vi "DigitalInput Reservations.vi"(3 "Reset":bool, 5 "Line":tag) -> (0 "Exit code":T1, 1 "Index assigned":i32, 2 "DigitalInput lines":tag[](array[tag]))   [LabVIEW 2015]
doc: "Attempt to reserve a line as a digital input. This also returns a list of lines that have been previously reserved.\n\nAs a Device developer, just call this with the line you want to add, check that the exit code is good, and save the assigned index.\n\nAs a Rack developer, remember to reset the reservations list before Device initialization and then call it with an empty line afterwards to get the list of digital output lines."
uses:
  Typedefs/Reservation exit codes.ctl
  <vilib>/Utility/error.llb/DialogType.ctl
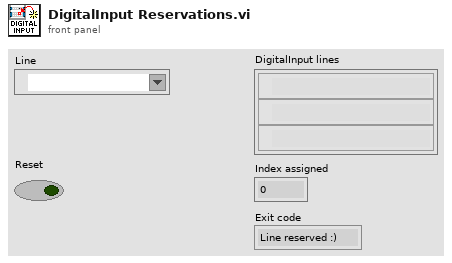
[diagram p1: front panel]
types:
  T1 = typedef "Reservation exit codes.ctl" = enum16{"Line reserved :)", "List reset.", "Empty line!", "Bad line!", "Already reserved!", "Timestamp conflict!", "Timestamp empty."}
  T2 = typedef "DialogType.ctl" = u16
  T3 = enum16{"Analog input", "Analog output", "Digital input", "Digital output", "Counter input", "Counter output"}
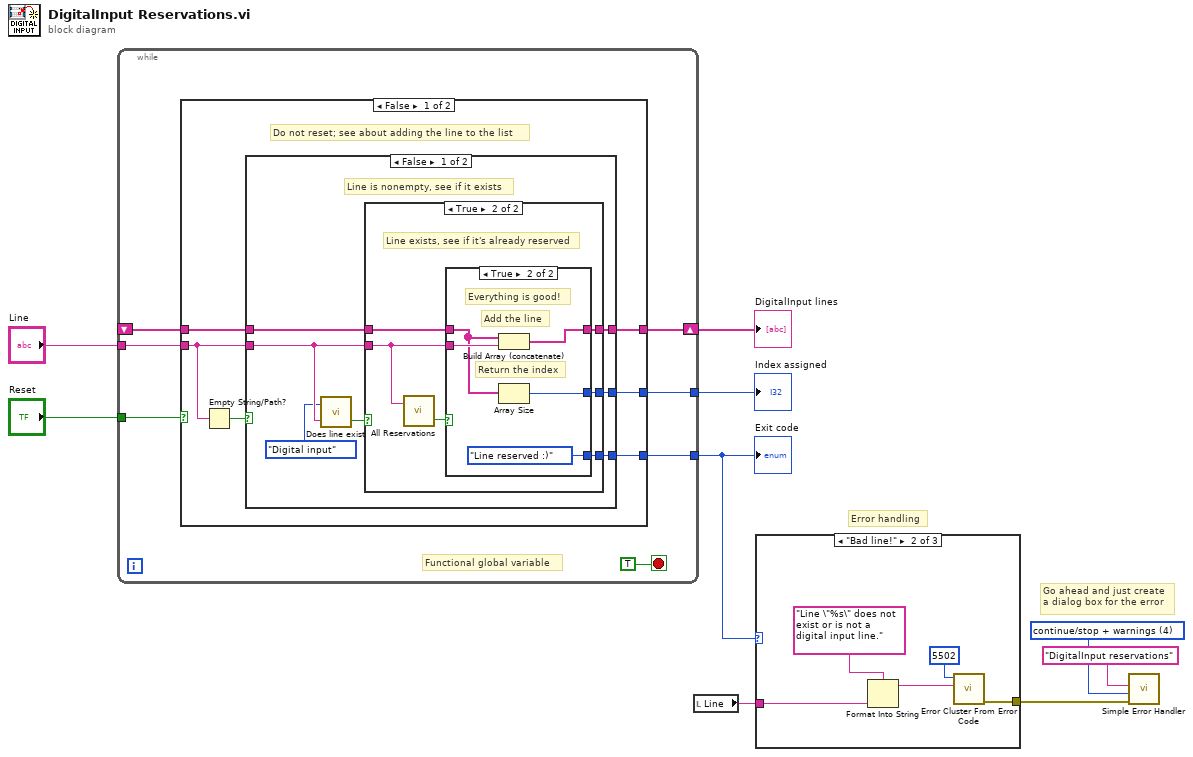
[diagram p0: block diagram]
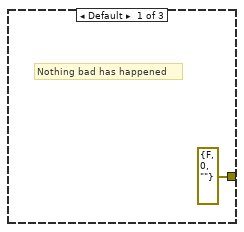
[diagram p2: hidden frame]
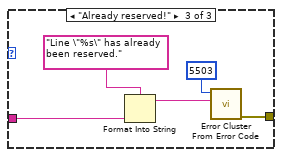
[diagram p3: hidden frame]
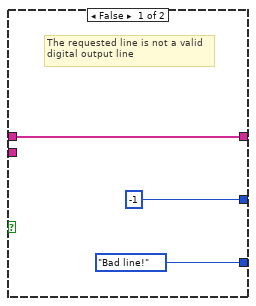
[diagram p4: hidden frame]
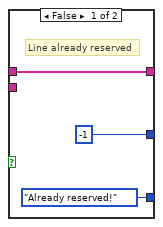
[diagram p5: hidden frame]
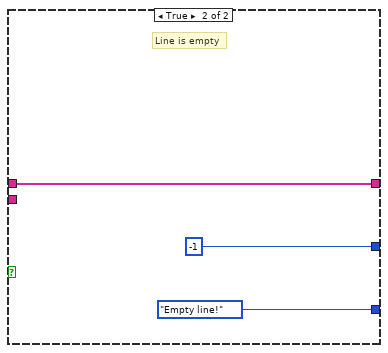
[diagram p6: hidden frame]
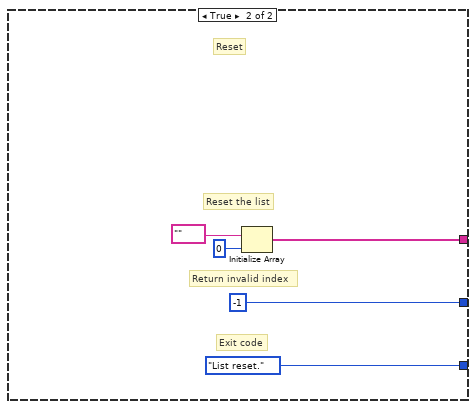
[diagram p7: hidden frame]
diagram:
  w4 = T2 4 items=["no dialog", "OK message", "continue or stop message", "OK message + warnings", "continue/stop + warnings"] ("type of dialog (OK msg:1)")
  # "Error handling"
  # "Go ahead and just create\na dialog box for the error"
  n1 = while {
    tunnel: [w16] -> w2
    tunnel: "Reset" -> [w15]
    shift-right: [w14] -> w9
    shift-left: _ -> [w12]
    tunnel: "Line" -> [w11]
    tunnel: [w10] -> w7
    stop <- TRUE ("stop") stop-if-true
    # "Functional global variable"
    n2 = case shown="False" w15 {
      tunnel: [w19 Reservation_exit_codes."List reset." ("Exit code")] -> w16
      tunnel: [w22 w53] -> w14
      tunnel: w12 -> [w21 _]
      tunnel: w11 -> [w17 _]
      tunnel: [w20 -1 ("Index assigned")] -> w10
      frame False {
        # "Do not reset; see about adding the line to the list"
        n3 = Empty String/Path?(string/path=w17) -> (empty?=w18:bool)
        n4 = case shown="False" w18 {
          tunnel: [w29 w49] -> w22
          tunnel: w21 -> [w28 w49]
          tunnel: [w27 -1] -> w20
          tunnel: [w26 Reservation_exit_codes."Empty line!" ("Exit code")] -> w19
          tunnel: w17 -> [w24 _]
          frame False {
            # "Line is nonempty, see if it exists"
            n5 = call "Does line exist.vi"("Line to look for"=w24, "Line type"=T3."Digital input") -> ("Does line exist?"=w25:bool)  [unwired: 1 out]
            n6 = case shown="True" w25 {
              tunnel: [w32 w38] -> w29
              tunnel: w28 -> [w32 w37]
              tunnel: [-1 w36] -> w27
              tunnel: [Reservation_exit_codes."Bad line!" ("Exit code") w35] -> w26
              tunnel: w24 -> [_ w33]
              frame False {
                # "The requested line is not a valid\ndigital output line"
              }
              frame True {
                # "Line exists, see if it's already reserved"
                n7 = call "All Reservations.vi"("Line to add"=w33) -> ("Line added?"=w34:bool)  [unwired: 1 in, 1 out]
                n8 = case shown="True" w34 {
                  tunnel: w37 -> [w41 w44]
                  tunnel: [w41 w46] -> w38
                  tunnel: w33 -> [_ w45]
                  tunnel: [-1 w43] -> w36
                  tunnel: [Reservation_exit_codes."Already reserved!" ("Exit code") Reservation_exit_codes."Line reserved :)" ("Exit code")] -> w35
                  frame False {
                    # "Line already reserved"
                  }
                  frame True {
                    # "Everything is good!"
                    # "Return the index"
                    # "Add the line"
                    n9 = Build Array (concatenate)(w44, w45) -> (w46:tag[])
                    n10 = Array Size(array=w44) -> (size(s)=w43:i32)
                  }
                }
              }
            }
          }
          frame True {
            # "Line is empty"
          }
        }
      }
      frame True {
        # "Reset"
        # "Exit code"
        # "Return invalid index"
        # "Reset the list"
        n11 = Initialize Array(tag "" ("Line to add"), 0 ("dimension size")) -> (w53:tag[])
      }
    }
  }
  "DigitalInput lines" <- w9
  "Exit code" <- w2
  "Index assigned" <- w7
  n12 = local read "Line"() -> (w1:tag)
  n13 = case shown="\"Bad line!\"" w2 {
    tunnel: w1 -> [_ w57 w61]
    tunnel: [errorcluster {"status"=FALSE, "code"=0, "source"=""} ("error out") w56 w62] -> w3
    frame Default {
      # "Nothing bad has happened"
    }
    frame "Bad line!" {
      n14 = Format Into String(format string="Line \"%s\" does not exist or is not a digital input line.", w57) -> (resulting string=w60:string)  [unwired: 2 in, 1 out]
      n15 = call <vilib>:"Error Cluster From Error Code.vi"("error message (\"\")"=w60, "error code (0)"=5502) -> ("error out"=w56:errorcluster)  [unwired: 7 in]
    }
    frame "Already reserved!" {
      n16 = Format Into String(format string="Line \"%s\" has already been reserved.", w61) -> (resulting string=w63:string)  [unwired: 2 in, 1 out]
      n17 = call <vilib>:"Error Cluster From Error Code.vi"("error message (\"\")"=w63, "error code (0)"=5503) -> ("error out"=w62:errorcluster)  [unwired: 7 in]
    }
  }
  n18 = call <vilib>:"Simple Error Handler.vi"("error source (\" \")"="DigitalInput reservations" ("error source (\" \")"), "type of dialog (OK msg:1)"=w4, "error in (no error)"=w3) -> ()  [unwired: 2 in, 5 out]
